vi "ResistanceToTemperature.vi"(1 "R_25":dbl=10000.0 format="%#_13g", 2 "Thermistor Resistance / Ohms":dbl=5000.0) -> (0 "Temperature / C":dbl=41.580344003974176 format="%0.2f")   [LabVIEW 2014]
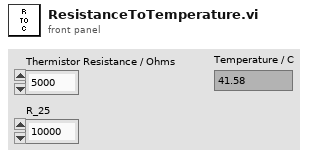
[diagram p1: front panel]
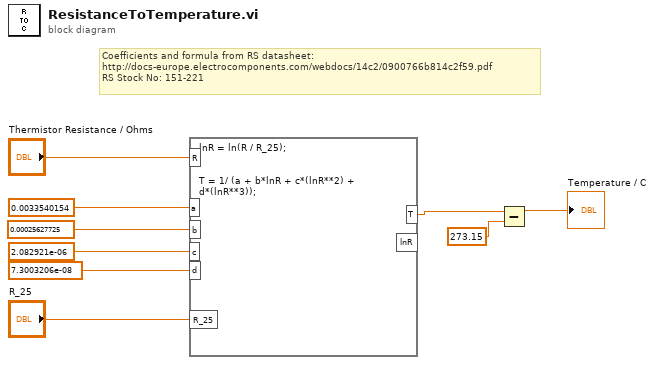
[diagram p0: block diagram]
diagram:
  # "Coefficients and formula from RS datasheet:\nhttp://docs-europe.electrocomponents.com/webdocs/14c2/0900766b814c2f59.pdf\nRS Stock No: 151-221"
  n1 = formula code="lnR = ln(R / R_25);\n\n\nT = 1/ (a + b*lnR + c*(lnR**2) + d*(lnR**3));"("a"=0.0033540154, "b"=0.00025627725, "c"=2.082921e-06, "R"="Thermistor Resistance / Ohms", "d"=7.3003206e-08 ("input variable"), "R_25"="R_25") -> ("T"=w9:dbl)  [unwired: 1 out]
  n2 = Subtract(x=w9, y=273.15) -> (x-y=→"Temperature / C":dbl)
